vi "Get Operating system.vi"(8 "error in (no error)":errorcluster, 11 "RT Management in":refnum<class "RT Management.lvclass">) -> (0 "error out":errorcluster, 2 "Operating system":T1, 3 "RT Management out":refnum<class "RT Management.lvclass">)   [LabVIEW 2015, in "RT Management.lvlib" / "RT Management.lvclass"]
uses:
  RT Management.lvclass
  Controls/Operating system.ctl
  RT Management.lvclass/RT Management.ctl
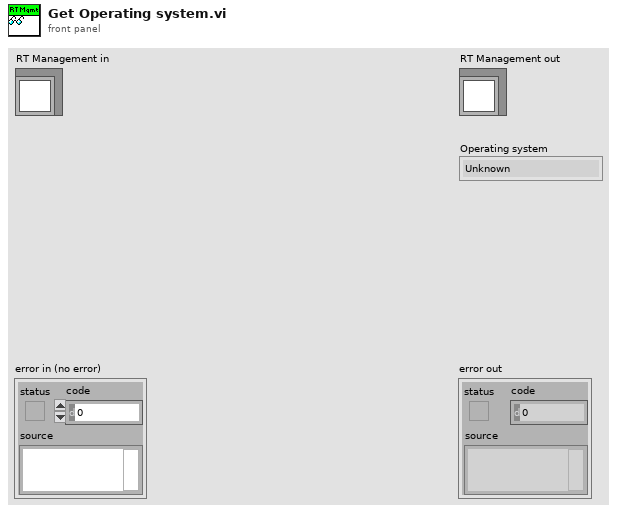
[diagram p1: front panel]
types:
  T1 = typedef "RT Management.lvlib/RT Management.lvclass/Operating system.ctl" = enum16{"Unknown", "VxWorks", "PharLap", "Linux-ARM", "Linux-x64"}
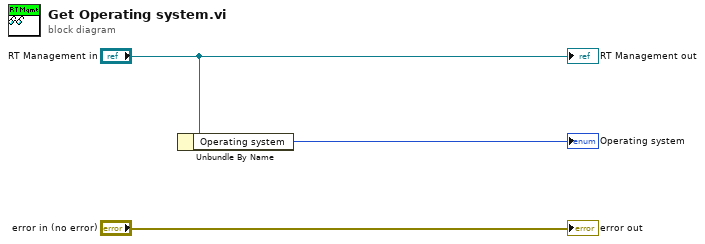
[diagram p0: block diagram]
diagram:
  n1 = Unbundle By Name("RT Management in") -> ("Operating system"=→"Operating system":T1)
  "error out" <- "error in (no error)"
  "RT Management out" <- "RT Management in"
